vi "State Checking.vi"(8 "error in (no error)":errorcluster, 10 "State Checking (T: On)":bool=TRUE, 11 "VISA resource name":refnum<visa-resource-name>) -> (0 "error out":errorcluster, 3 "VISA resource name out":refnum<visa-resource-name>)   [LabVIEW 2014, in "Fluke 5XXX Series Multicalibrators.lvlib"]
doc: "This VI switches state checking of the instrument (reading of the Standard Event Register and checking it for error) status subsystem. Driver VIs are using state checking which is by default enabled.\n\nNote:\n\n(1) In debug mode enable state checking.\n\n(2) For better bus throughput and instruments performance disable state checking.\n\n(3) When state checking is disabled driver does not check if correct instrument model or option is used with each of the VIs. This might cause unexpected behaviour of the instrument.\n\n(4) Simpliest way how to disable state checking from the begining is calling initialization VI with the parameter ID Query = False. But this is not recommended as functionality of the driver depends on the instrument model and its options."
uses:
  Fluke 5XXX Series Multicalibrators.lvlib
panel:
  # "On"
  # "Off"
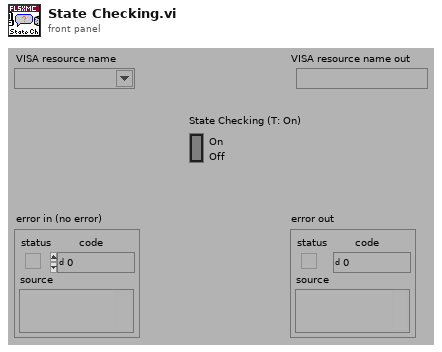
[diagram p1: front panel]
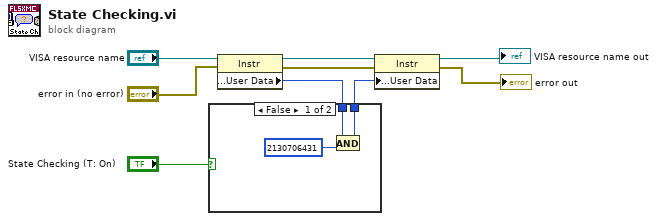
[diagram p0: block diagram]
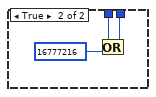
[diagram p2: hidden frame]
diagram:
  n1 = property class="Instr"(reference="VISA resource name", error in="error in (no error)") -> (reference out=w6:refnum<visa-resource-name>, error out=w5:errorcluster, "General Settings:User Data"=w3:u32)
  n2 = case shown="False" "State Checking (T: On)" {
    tunnel: w3 -> [w12 w15]
    tunnel: [w11 w14] -> w2
    frame False {
      n3 = And(x=w12, y=u32 2130706431 (".not. (x .and. y)?")) -> (x .and. y?=w11:u32)
    }
    frame True {
      n4 = Or(x=w15, y=u32 16777216 (".not. (x .and. y)?")) -> (x .or. y?=w14:u32)
    }
  }
  n5 = property class="Instr"(reference=w6, error in=w5, "General Settings:User Data"=w2) -> (reference out=→"VISA resource name out":refnum<visa-resource-name>, error out=→"error out":errorcluster)
